vi "Launch UI.vi"(8 "error in (no error)":errorcluster, 11 "Controller in":refnum<class "Controller.lvclass">) -> (0 "error out":errorcluster, 3 "Controller out":refnum<class "Controller.lvclass">)   [LabVIEW 2022 SP3, in "Controller.lvlib" / "Controller.lvclass"]
uses:
  Controller.lvclass
  C:/Program Files/National Instruments/LabVIEW 2022/vi.lib/ActorFramework/Actor/Actor.lvclass
  UserInterface/UserInterface/UserInterface.lvclass
  Controller.lvclass/Controller.ctl
  <vilib>/ActorFramework/Actor/Actor.lvclass
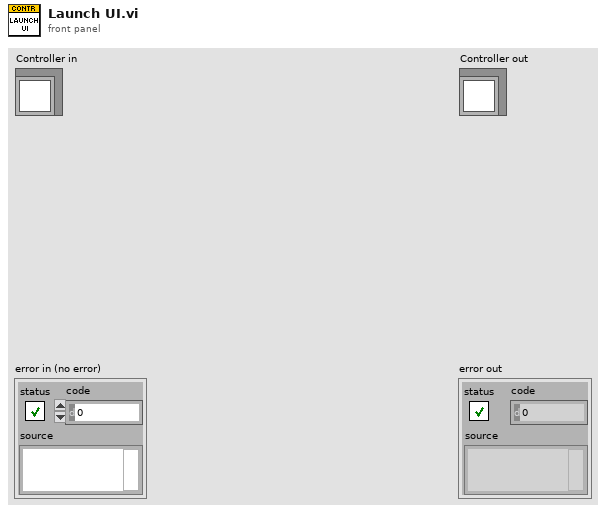
[diagram p1: front panel]
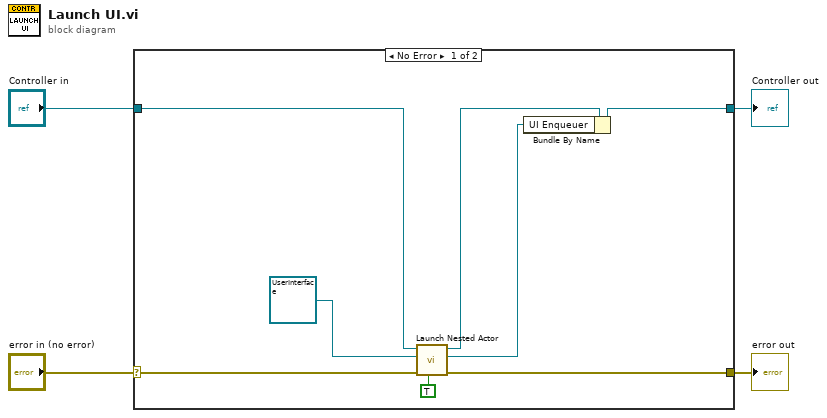
[diagram p0: block diagram]
diagram:
  n1 = case shown="No Error" "error in (no error)" {
    selector: "error in (no error)" -> [w12 w14]
    tunnel: [w11 w14] -> w3
    tunnel: [w6 w13] -> w1
    tunnel: "Controller in" -> [w10 w13]
    frame No Error {
      n2 = call <vilib>:"Launch Nested Actor.vi"("Open Actor Core front panel? (F)"=TRUE, "error in (no error)"=w12, "Nested Actor"=refnum<class "UserInterface.lvclass"> refnum ("UserInterface.lvlib:UserInterface.lvclass"), "Caller Actor in"=w10) -> ("error out"=w11:errorcluster, "Nested Actor's Enqueuer"=w5:refnum<class "Message Enqueuer.lvclass">, "Caller Actor out"=w9:refnum<class "Controller.lvclass">)  [unwired: 5 in]
      n3 = Bundle By Name(cluster=w9, "UI Enqueuer"=w5) -> (w6:refnum<class "Controller.lvclass">)
    }
    frame Error {
    }
  }
  "error out" <- w3
  "Controller out" <- w1
